vi "Untitled 3.vi"() -> ()   [LabVIEW 2019]
panel:
  out "Tip Position":dbl[](array[numeric])
  out "Z":dbl
  out "Y":dbl
  in  "Radius":dbl
  out "alpha":dbl
  in  "degree":dbl
  in  "Numeric":dbl
  out "kt":dbl
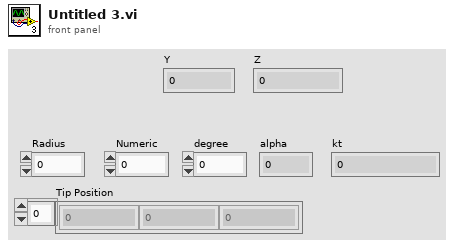
[diagram p1: front panel]
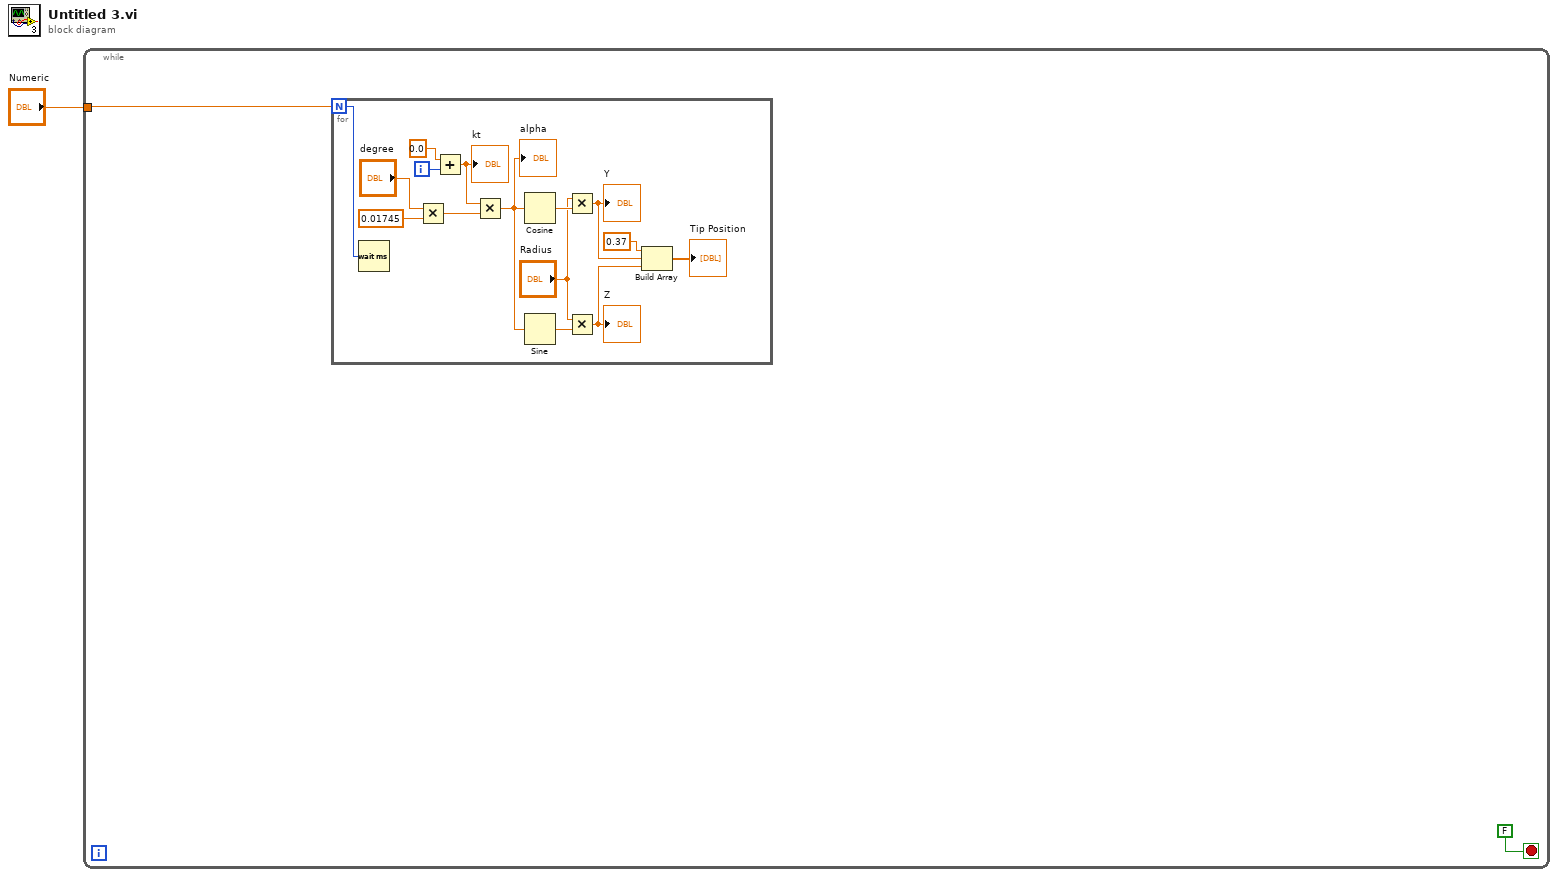
[diagram p0: block diagram]
diagram:
  n1 = while {
    tunnel: "Numeric" -> [w2]
    stop <- FALSE stop-if-true
    n2 = for {
      N: w2 -> [w17]
      i -> [w18]
      n3 = Wait (ms)(milliseconds to wait=w17) -> ()  [unwired: 1 out]
      n4 = Multiply(x="degree", y=0.01745) -> (x*y=w12:dbl)
      n5 = Add(x=0.0 ("startValue"), y=w18) -> (x+y=w15:dbl)
      "kt" <- w15
      n6 = Multiply(x=w15, y=w12) -> (x*y=w10:dbl)
      "alpha" <- w10
      n7 = Cosine(x=w10) -> (cos(x)=w11:dbl)
      n8 = Sine(x=w10) -> (sin(x)=w8:dbl)
      n9 = Multiply(x="Radius", y=w11) -> (x*y=w6:dbl)
      "Y" <- w6
      n10 = Multiply(x="Radius", y=w8) -> (x*y=w5:dbl)
      "Z" <- w5
      n11 = Build Array(0.37, w6, w5) -> (→"Tip Position":dbl[])
    }
  }
